vi "Query_Tree_PN.vi"(2 "Trimmed down TreeNode array":T1[](array[typedef]), 3 "Query Y":dbl, 4 "Query X":dbl) -> (0 "Indices of traversed treenodes":i32[](array[numeric]), 1 "Indices of triangle array to test fully":i32[](array[numeric]))   [LabVIEW 2010]
uses:
  Trimmed down TreeNode2D.ctl
panel:
  # "Paul Nathan 05/03/10\n\n09/03/10: Modified to use\ntrimmed down treenode array\nfor speed"
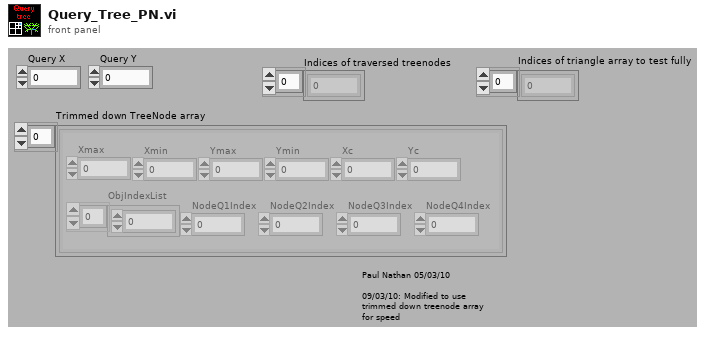
[diagram p1: front panel]
types:
  T1 = typedef "Trimmed down TreeNode2D.ctl" = cluster{"Xmax":dbl, "Xmin":dbl, "Ymax":dbl, "Ymin":dbl, "Xc":dbl, "Yc":dbl, "ObjIndexList":i32[], "NodeQ1Index":i32, "NodeQ2Index":i32, "NodeQ3Index":i32, "NodeQ4Index":i32}
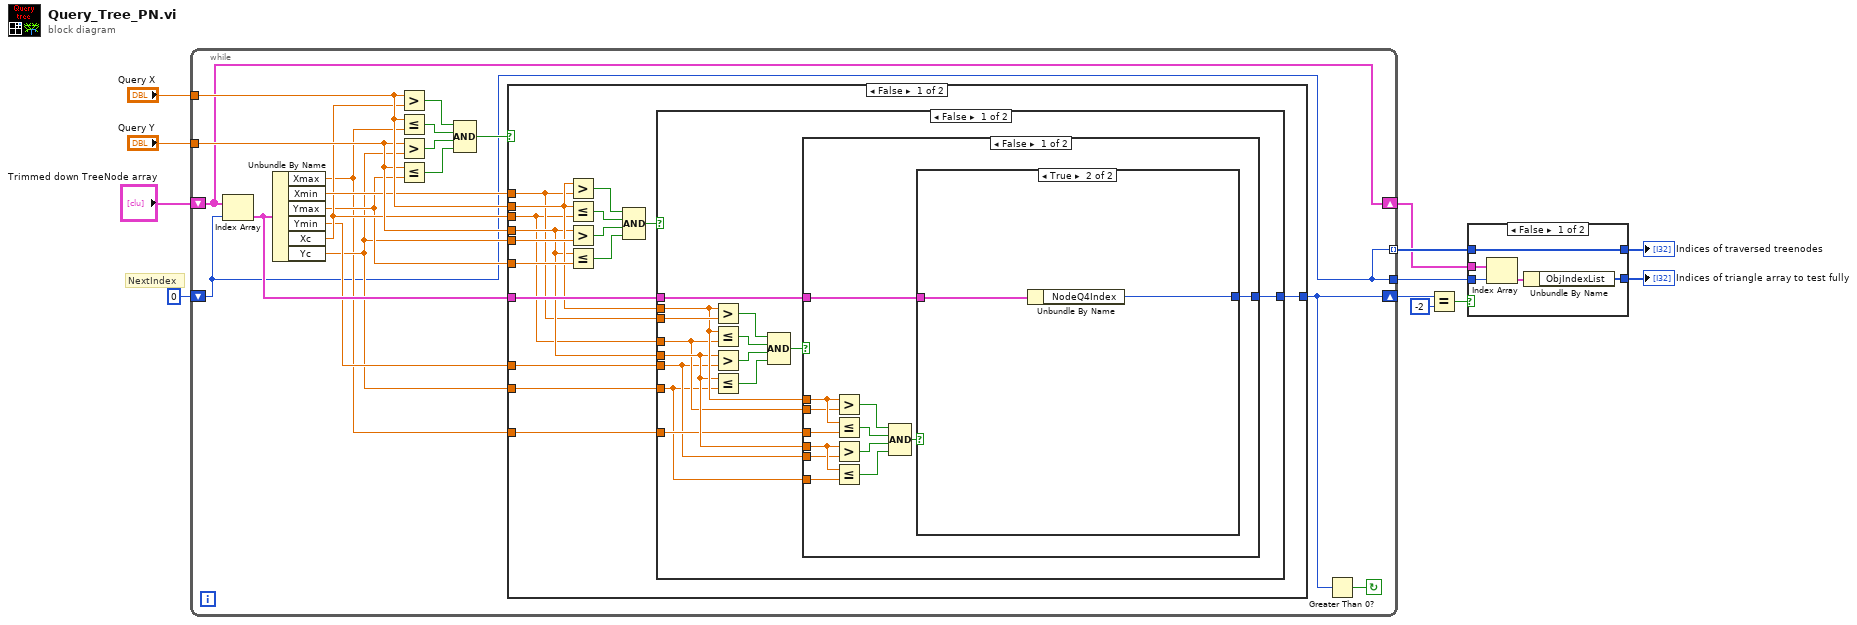
[diagram p0: block diagram]
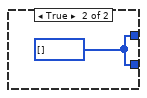
[diagram p2: hidden frame]
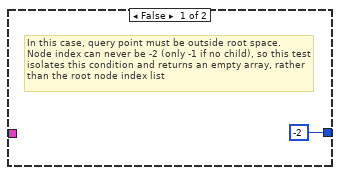
[diagram p3: hidden frame]
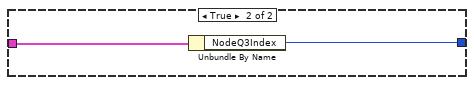
[diagram p4: hidden frame]
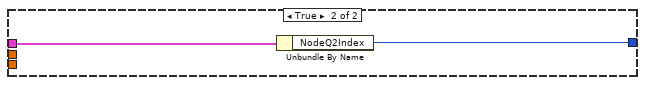
[diagram p5: hidden frame]
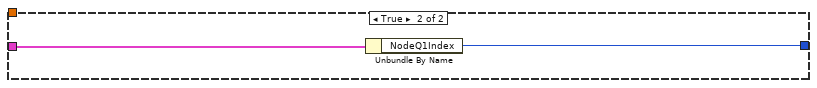
[diagram p6: hidden frame]
diagram:
  # "NextIndex"
  n1 = while {
    tunnel: "Query X" -> [w23]
    tunnel: "Query Y" -> [w22]
    shift-right: [w15] -> w10
    shift-left: 0 -> [w14]
    tunnel: [w14] -> w4
    tunnel: [w14] -> w5 mode=indexing
    shift-right: [w13] -> w2
    shift-left: "Trimmed down TreeNode array" -> [w13]
    stop <- w30 continue-if-true
    n2 = Index Array(array=w13, index=w14) -> (element=w24:T1)
    n3 = Unbundle By Name(w24) -> ("Xmax"=w16:dbl, "Xmin"=w21:dbl, "Ymax"=w19:dbl, "Ymin"=w18:dbl, "Xc"=w20:dbl, "Yc"=w17:dbl)
    n4 = Greater?(x=w23, y=w20) -> (0:w29:bool)
    n5 = Less Or Equal?(x=w23, y=w16) -> (x <= y?=w28:bool)
    n6 = Greater?(x=w22, y=w17) -> (0:w27:bool)
    n7 = Less Or Equal?(x=w22, y=w19) -> (x <= y?=w26:bool)
    n8 = Compound Arithmetic op=AND(w29, w28, w27, w26) -> (w25:bool)
    n9 = case shown="False" w25 {
      tunnel: w24 -> [w40 w82]
      tunnel: [w39 w81] -> w15
      tunnel: w23 -> [w37 _]
      tunnel: w22 -> [w36 _]
      tunnel: w21 -> [w35 _]
      tunnel: w20 -> [w34 _]
      tunnel: w17 -> [w42 _]
      tunnel: w19 -> [w41 _]
      tunnel: w18 -> [w33 _]
      tunnel: w17 -> [w32 _]
      tunnel: w16 -> [w31 _]
      frame False {
        n10 = Greater?(x=w37, y=w35) -> (0:w43:bool)
        n11 = Less Or Equal?(x=w37, y=w34) -> (x <= y?=w44:bool)
        n12 = Greater?(x=w36, y=w42) -> (0:w45:bool)
        n13 = Less Or Equal?(x=w36, y=w41) -> (x <= y?=w46:bool)
        n14 = Compound Arithmetic op=AND(w43, w44, w45, w46) -> (w38:bool)
        n15 = case shown="False" w38 {
          tunnel: w40 -> [w48 w80]
          tunnel: [w47 w79] -> w39
          tunnel: w37 -> [w54 _]
          tunnel: w36 -> [w53 _]
          tunnel: w35 -> [w56 _]
          tunnel: w34 -> [w52 _]
          tunnel: w33 -> [w50 _]
          tunnel: w32 -> [w49 _]
          tunnel: w31 -> [w51 _]
          frame False {
            n16 = Greater?(x=w54, y=w56) -> (0:w60:bool)
            n17 = Less Or Equal?(x=w54, y=w52) -> (x <= y?=w59:bool)
            n18 = Greater?(x=w53, y=w50) -> (0:w58:bool)
            n19 = Less Or Equal?(x=w53, y=w49) -> (x <= y?=w57:bool)
            n20 = Compound Arithmetic op=AND(w60, w59, w58, w57) -> (w55:bool)
            n21 = case shown="False" w55 {
              tunnel: w54 -> [w69 _]
              tunnel: w53 -> [w68 _]
              tunnel: w52 -> [w67 _]
              tunnel: w51 -> [w66 _]
              tunnel: w50 -> [w65 _]
              tunnel: w49 -> [w64 _]
              tunnel: w48 -> [w62 w78]
              tunnel: [w61 w77] -> w47
              frame False {
                n22 = Greater?(x=w69, y=w67) -> (0:w70:bool)
                n23 = Less Or Equal?(x=w69, y=w66) -> (x <= y?=w71:bool)
                n24 = Greater?(x=w68, y=w65) -> (0:w72:bool)
                n25 = Less Or Equal?(x=w68, y=w64) -> (x <= y?=w73:bool)
                n26 = Compound Arithmetic op=AND(w70, w71, w72, w73) -> (w63:bool)
                n27 = case shown="True" w63 {
                  tunnel: w62 -> [_ w76]
                  tunnel: [-2 ("NodeQ4Index") w75] -> w61
                  frame False {
                    # "In this case, query point must be outside root space.\nNode index can never be -2 (only -1 if no child), so this test isolates this condition and returns an empty array, rather than the root node index list"
                  }
                  frame True {
                    n28 = Unbundle By Name(w76) -> ("NodeQ4Index"=w75:i32)
                  }
                }
              }
              frame True {
                n29 = Unbundle By Name(w78) -> ("NodeQ3Index"=w77:i32)
              }
            }
          }
          frame True {
            n30 = Unbundle By Name(w80) -> ("NodeQ2Index"=w79:i32)
          }
        }
      }
      frame True {
        n31 = Unbundle By Name(w82) -> ("NodeQ1Index"=w81:i32)
      }
    }
    n32 = Greater Than 0?(x=w15) -> (x > 0?=w30:bool)
  }
  n33 = Equal?(x=w10, y=-2) -> (x = y?=w8:bool)
  n34 = case shown="False" w8 {
    tunnel: [w83 w88] -> w7
    tunnel: [w84 w88] -> w6
    tunnel: w5 -> [w84 _]
    tunnel: w4 -> [w85 _]
    tunnel: w2 -> [w86 _]
    frame False {
      n35 = Index Array(array=w86, index=w85) -> (element=w87:T1)
      n36 = Unbundle By Name(w87) -> ("ObjIndexList"=w83:i32[])
    }
    frame True {
      w88 = i32[] [] ("ObjIndexList")
    }
  }
  "Indices of triangle array to test fully" <- w7
  "Indices of traversed treenodes" <- w6
